vi "destroyReferencesTwoTcpServers.vi"(8 "error in (no error)":errorcluster, 11 "TcpServer in":refnum<class "TcpServer.lvclass">) -> (0 "error out":errorcluster, 3 "TcpServer out":refnum<class "TcpServer.lvclass">)   [LabVIEW 2018]
doc: "Release notifier references and unregister user events references for Cmd and Tel instances of TcpServer."
uses:
  src/TcpServer/TcpServer.lvclass
  src/TcpServer/TcpServer.lvclass/TcpServer.ctl
  src/TcpServerTel/TcpServerTel.lvclass/TcpServerTel.ctl
  src/TcpServerCmd/TcpServerCmd.lvclass
  home/pcortes/Documents/github/ts_labview_tcp_json/src/TcpServerBase/TcpServerBase.lvclass
  src/TcpServerTel/TcpServerTel.lvclass
  src/TcpServerBase/TcpServerBase.lvclass
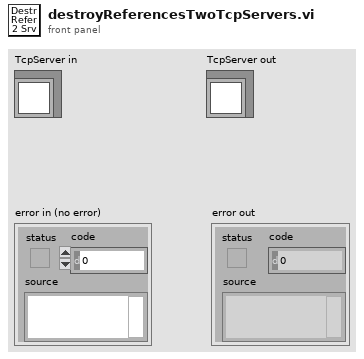
[diagram p1: front panel]
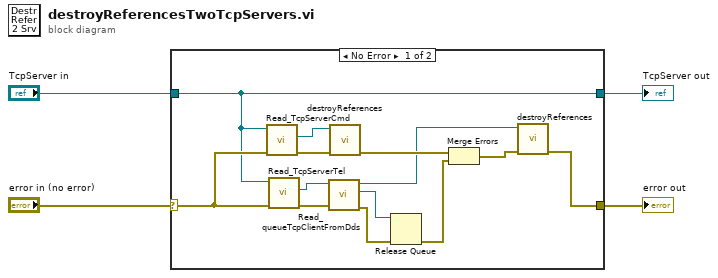
[diagram p0: block diagram]
diagram:
  n1 = case shown="No Error" "error in (no error)" {
    selector: "error in (no error)" -> [w13 w18]
    tunnel: [w12 w18] -> w3
    tunnel: "TcpServer in" -> [w11 w19]
    tunnel: [w11 w19] -> w1
    frame No Error {
      n2 = call "Read_TcpServerCmd.vi"("error in (no error)"=w13, "TcpServer in"=w11) -> ("error out"=w15:errorcluster, "TcpServerCmd.lvclass"=w14:refnum<class "TcpServerCmd.lvclass">)  [unwired: 7 in, 1 out]
      n3 = call "Read_TcpServerTel.vi"("error in (no error)"=w13, "TcpServer in"=w11) -> ("error out"=w7:errorcluster, "TcpServerTel.lvclass"=w8:refnum<class "TcpServerTel.lvclass">)  [unwired: 7 in, 1 out]
      n4 = call "Read_queueTcpClientFromDds.vi"("error in (no error)"=w7, "TcpServerTel in"=w8) -> ("error out"=w10:errorcluster, "queueTcpClientFromDds"=w9:refnum<queue>, "TcpServerTel out"=w6:refnum<class "TcpServerTel.lvclass">)  [unwired: 7 in]
      n5 = call "destroyReferences.vi"("error in (no error)"=w15, "tcpServerBase in"=w14) -> ("error out"=w16:errorcluster)  [unwired: 8 in, 1 out]
      n6 = Release Queue(queue=w9, error in (no error)=w10) -> (error out=w5:errorcluster)  [unwired: 1 in, 2 out]
      n7 = Merge Errors(w16, w5) -> (w17:errorcluster)
      n8 = call "destroyReferences.vi"("error in (no error)"=w17, "tcpServerBase in"=w6) -> ("error out"=w12:errorcluster)  [unwired: 8 in, 1 out]
    }
    frame Error {
    }
  }
  "error out" <- w3
  "TcpServer out" <- w1
